vi "Read Wheel State.vi"(8 "error in (no error)":errorcluster, 10 "wheel state in":T1, 11 "caster wheel in":refnum<class "NI_Robotics_Caster Wheel.lvclass">) -> (0 "error out":errorcluster, 2 "wheel state out":T1, 3 "caster wheel out":refnum<class "NI_Robotics_Caster Wheel.lvclass">)   [LabVIEW 2017, in "NI_Robotics_Caster Wheel.lvclass"]
uses:
  <vilib>/robotics/Steering/Caster Wheel/NI_Robotics_Caster Wheel.lvclass
  <vilib>/robotics/Steering/Wheel/Wheel State.ctl
  <vilib>/robotics/Steering/Caster Wheel/NI_Robotics_Caster Wheel.lvclass/NI_Robotics_Caster Wheel.ctl
  <vilib>/robotics/Actuation/Motor Communication/Get Motor Velocity State.vi
  <vilib>/robotics/Actuation/Motor Communication/Get Motor Angle State.vi
  <vilib>/robotics/Actuation/Motor Communication/Check if Valid.vi
  <vilib>/robotics/Utilities/Generate Error.vi
  <vilib>/robotics/Steering/Wheel/NI_Robotics_Wheel.lvclass
  <vilib>/robotics/Actuation/Motor Communication/NI_Robotics_Motor Communication.lvclass
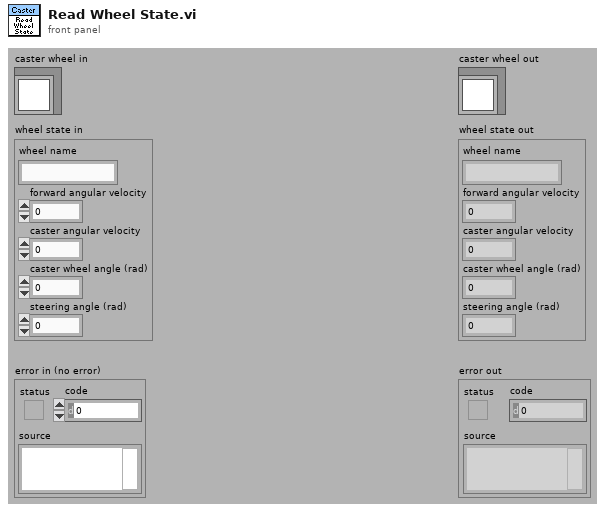
[diagram p1: front panel]
types:
  T1 = typedef "NI_Robotics_Wheel.lvclass/Wheel State.ctl" = cluster{"wheel name":string, "forward angular velocity":dbl, "caster angular velocity":dbl, "caster wheel angle (rad)":dbl, "steering angle (rad)":dbl}
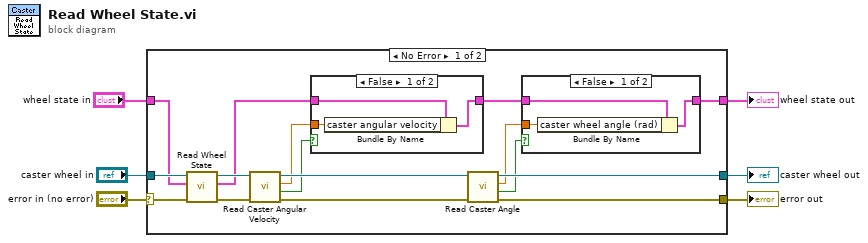
[diagram p0: block diagram]
diagram:
  n1 = case shown="No Error" "error in (no error)" {
    selector: "error in (no error)" -> [w21 w32]
    tunnel: [w15 w32] -> w6
    tunnel: [w7 w31] -> w5
    tunnel: [w16 w33] -> w4
    tunnel: "caster wheel in" -> [w22 w33]
    tunnel: "wheel state in" -> [w14 w31]
    frame No Error {
      n2 = call-parent "Read Wheel State.vi"("error in (no error)"=w21, "wheel state in"=w14, "wheel in"=w22) -> ("error out"=w19:errorcluster, "wheel state out"=w12:T1, "wheel out"=w20:refnum<class "NI_Robotics_Caster Wheel.lvclass">)  [unwired: 6 in]
      n3 = call <vilib>:"Read Caster Angular Velocity.vi"("error in (no error)"=w19, "caster wheel in"=w20) -> ("error out"=w17:errorcluster, "failed"=w11:bool, "caster angular velocity"=w13:dbl, "caster wheel out"=w18:refnum<class "NI_Robotics_Caster Wheel.lvclass">)  [unwired: 6 in]
      n4 = case shown="False" w11 {
        tunnel: w13 -> [w29 _]
        tunnel: w12 -> [w28 w30]
        tunnel: [w27 w30] -> w10
        frame False {
          n5 = Bundle By Name(cluster=w28, "caster angular velocity"=w29) -> (w27:T1)
        }
        frame True {
        }
      }
      n6 = call <vilib>:"Read Caster Angle.vi"("error in (no error)"=w17, "caster wheel in"=w18) -> ("error out"=w15:errorcluster, "failed"=w8:bool, "caster angle (rad)"=w9:dbl, "caster wheel out"=w16:refnum<class "NI_Robotics_Caster Wheel.lvclass">)  [unwired: 6 in]
      n7 = case shown="False" w8 {
        tunnel: w9 -> [w25 _]
        tunnel: w10 -> [w24 w26]
        tunnel: [w23 w26] -> w7
        frame False {
          n8 = Bundle By Name(cluster=w24, "caster wheel angle (rad)"=w25) -> (w23:T1)
        }
        frame True {
        }
      }
    }
    frame Error {
    }
  }
  "error out" <- w6
  "caster wheel out" <- w4
  "wheel state out" <- w5
